vi "NumberToASCII.vi"(1 "number":i32) -> (0 "ASCII":string)   [LabVIEW 2012]
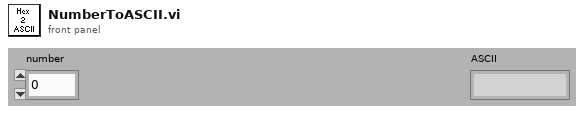
[diagram p1: front panel]
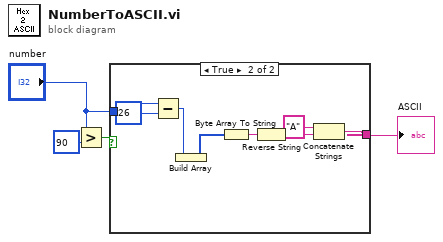
[diagram p0: block diagram]
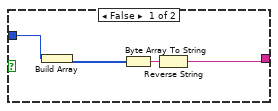
[diagram p2: hidden frame]
diagram:
  n1 = Greater?(x="number", y=90) -> (0:w2:bool)
  n2 = case shown="True" w2 {
    tunnel: [w5 w9] -> w4
    tunnel: "number" -> [w6 w14]
    frame False {
      n3 = Build Array(w6) -> (w7:i32[])
      n4 = Byte Array To String(unsigned byte array=w7) -> (string=w8:string)
      n5 = Reverse String(1:w8) -> (0:w5:string)
    }
    frame True {
      n6 = Subtract(x=w14, y=26) -> (x-y=w12:i32)
      n7 = Build Array(w12) -> (w15:i32[])
      n8 = Byte Array To String(unsigned byte array=w15) -> (string=w16:string)
      n9 = Reverse String(1:w16) -> (0:w11:string)
      n10 = Concatenate Strings("A" ("string"), w11) -> (w9:string)
    }
  }
  "ASCII" <- w4
